vi "HRM-common-send_status.vi"(7 "Module name":string, 8 "error in (no error)":errorcluster, 11 "init cluster":T1) -> (0 "error out":errorcluster)   [LabVIEW 2020]
uses:
  init/HRM-init-cluster.ctl
  init/HRM-init-user_events.ctl
  init/HRM-init-start_state.ctl
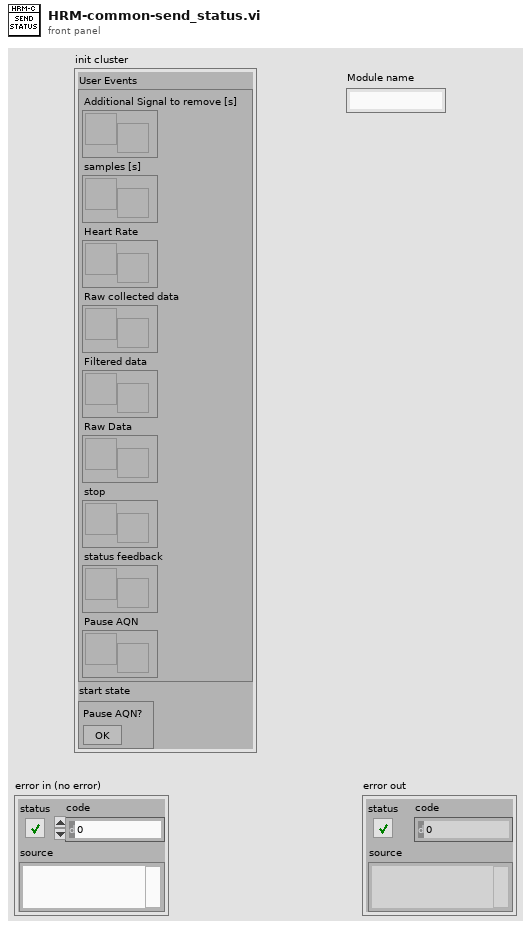
[diagram p1: front panel]
types:
  T1 = typedef "HRM-init-cluster.ctl" = cluster{"User Events":T2, "start state":T3}
  T2 = typedef "HRM-init-user_events.ctl" = cluster{"Additional Signal to remove [s]":refnum<user-event>, "samples [s]":refnum<user-event>, "Heart Rate":refnum<user-event>, "Raw collected data":refnum<user-event>, "Filtered data":refnum<user-event>, "Raw Data":refnum<user-event>, "stop":refnum<user-event>, "status feedback":refnum<user-event>, "Pause AQN":refnum<user-event>}
  T3 = typedef "HRM-init-start_state.ctl" = cluster{"Pause AQN?":bool}
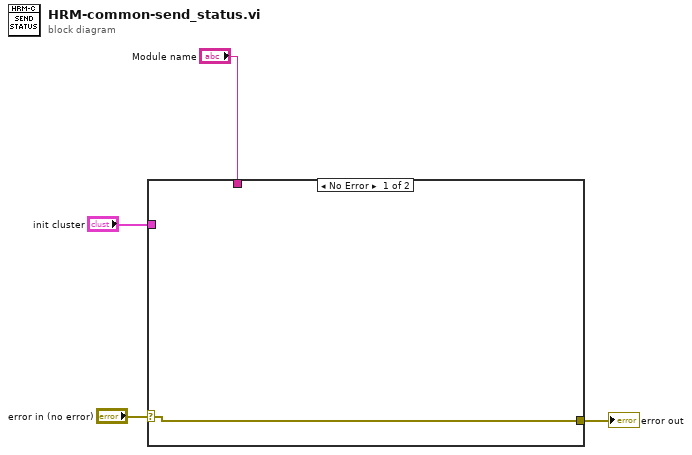
[diagram p0: block diagram]
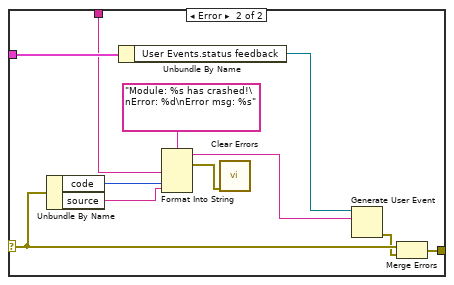
[diagram p2: hidden frame]
diagram:
  n1 = case shown="No Error" "error in (no error)" {
    selector: "error in (no error)" -> [w5 w8]
    tunnel: "init cluster" -> [_ w16]
    tunnel: "Module name" -> [_ w13]
    tunnel: [w5 w6] -> w1
    frame No Error {
    }
    frame Error {
      n2 = Unbundle By Name(w8) -> ("code"=w12:i32, "source"=w11:string)
      n3 = Unbundle By Name(w16) -> ("User Events.status feedback"=w15:refnum<user-event>)
      n4 = Format Into String(format string="Module: %s has crashed!\nError: %d\nError msg: %s", w13, w12, w11) -> (resulting string=w10:string, error out=w9:errorcluster)  [unwired: 2 in]
      n5 = call <vilib>:"Clear Errors.vi"("error in (no error)"=w9) -> ()  [unwired: 5 in, 2 out]
      n6 = Generate User Event(user event=w15, event data cluster=w10) -> (error out=w7:errorcluster)  [unwired: 2 in, 1 out]
      n7 = Merge Errors(w8, w7) -> (w6:errorcluster)
    }
  }
  "error out" <- w1
